vi "Motor_Temp_Monitor_V15.vi"() -> ()   [LabVIEW 2019]
uses:
  Instance           2 30Saved   Motor_Temp_Monitor_V11 .vi
  <vilib>/Utility/error.llb/DialogType.ctl
  Controls/Measurement Action.ctl
  <vilib>/ULx/Create Channel.llb/ULx Create Channel (DO-Digital Output).vi
  <vilib>/ULx/Write.llb/ULx Write (Digital Bool 1Line 1Point).vi
panel:
  out "Log Write":bool
  out "Cluster":T1 {"1" format="%.1f"; "11" format="%.1f"; "6" format="%.1f"; "9" format="%.1f"; "10" format="%.1f"; "15" format="%.1f"; "14" format="%.1f"; "13" format="%.1f"; "12" format="%.1f"; "5" format="%.1f"; "8" format="%.1f"; "2" format="%.1f"; "3" format="%.1f"; "4" format="%.1f"; "7" format="%.1f"}
  out "Stop Signal Status":bool
  in  "OK Button":bool
  out "Alarm":bool
  out "Alarm":bool
  in  "Motor Temp.\nLimit °C":sgl=60.0 min=0 max=200 step=1
  out "Time":string
  out "Date":string
  in  "Bearing Temp.\nLimit °C":sgl=40.0 min=0 max=200 step=1
  in  "stop":bool
  out "MOTOR TEMPERATURES\n[Deg C]":T2 caption="Motor Temperatures °C" {"6. Rear Motor: Armature Com End" format="%.1f"; "5. Rear Motor: Field Windings" format="%.1f"; "4. Rear Motor: Armature Ctr. Brg" format="%.1f"; "3. Front Motor: Armature Ctr. Brg" format="%.1f"; "1" format="%.1f"; "2\n2" format="%.1f"}
  in  "Tab Control":T3(tab)
  out "Motor Thermocouple Chart":waveform(dbl)[](graph)
  out "Motor Bearing Chart":waveform(dbl)[](graph)
  # "DOWTY PROPELLERS - WIND TUNNEL MOTOR TEMPERATURE MONITORING SYSTEM"
  # "V15.1 Ó2014 GE Aviation"
  # "M4"
  # "Motor Temperatures °C"
  # "M1"
  # "M2"
  # "M3"
  # "M4"
  # "M5"
  # "M6"
  # "2"
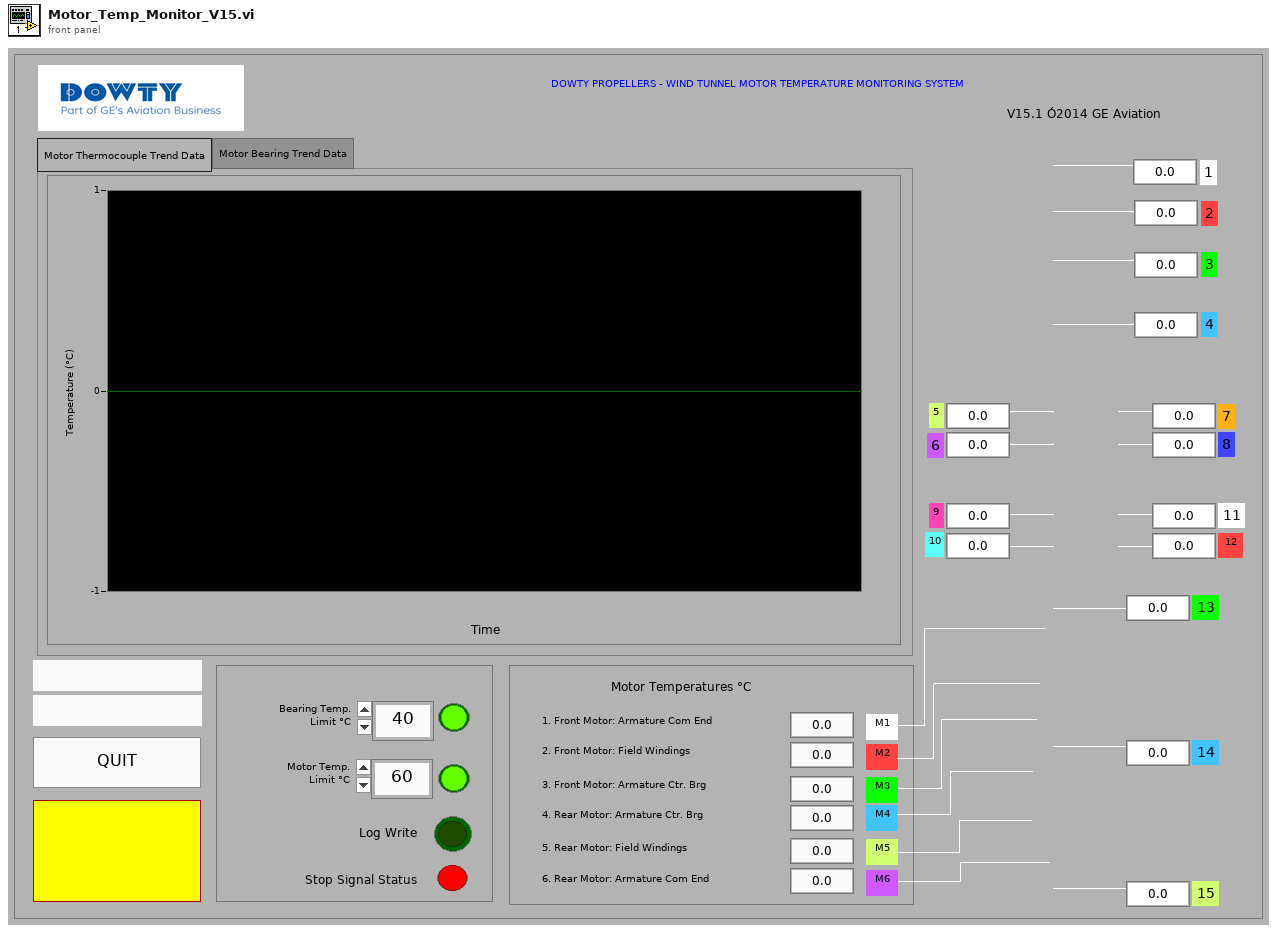
[diagram p1: front panel]
types:
  T1 = cluster{"1":sgl, "2":sgl, "3":sgl, "4":sgl, "5":sgl, "6":sgl, "7":sgl, "8":sgl, "9":sgl, "10":sgl, "11":sgl, "12":sgl, "13":sgl, "14":sgl, "15":sgl}
  T2 = cluster{"1":sgl, "2\n2":sgl, "3. Front Motor: Armature Ctr. Brg":sgl, "4. Rear Motor: Armature Ctr. Brg":sgl, "5. Rear Motor: Field Windings":sgl, "6. Rear Motor: Armature Com End":sgl}
  T3 = enum32{"Motor Thermocouple Trend Data", "Motor Bearing Trend Data"}
  T4 = typedef "Measurement Action.ctl" = enum16{"Open", "Read Bearing Temps", "Read Motor Temps", "Close"}
  T5 = enum16{"open", "replace", "create", "open or create", "replace or create", "replace or create with confirmation"}
  T6 = cluster{"second":i32, "minute":i32, "hour":i32, "day of month":i32, "month":i32, "year":i32, "day of week":i32, "day of year":i32, "is DST":i32}
  T7 = typedef "DialogType.ctl" = u16
  T8 = cluster{"Temps[0]":dbl, "Temps[1]":dbl, "Temps[2]":dbl, "Temps[3]":dbl, "Temps[4]":dbl, "Temps[5]":dbl}
  T9 = cluster{"Temps[0]":dbl, "Temps[1]":dbl, "Temps[2]":dbl, "Temps[3]":dbl, "Temps[4]":dbl, "Temps[5]":dbl, "Temps[6]":dbl, "Temps[7]":dbl, "Temps[8]":dbl, "Temps[9]":dbl, "Temps[10]":dbl, "Temps[11]":dbl, "Temps[12]":dbl, "Temps[13]":dbl, "Temps[14]":dbl}
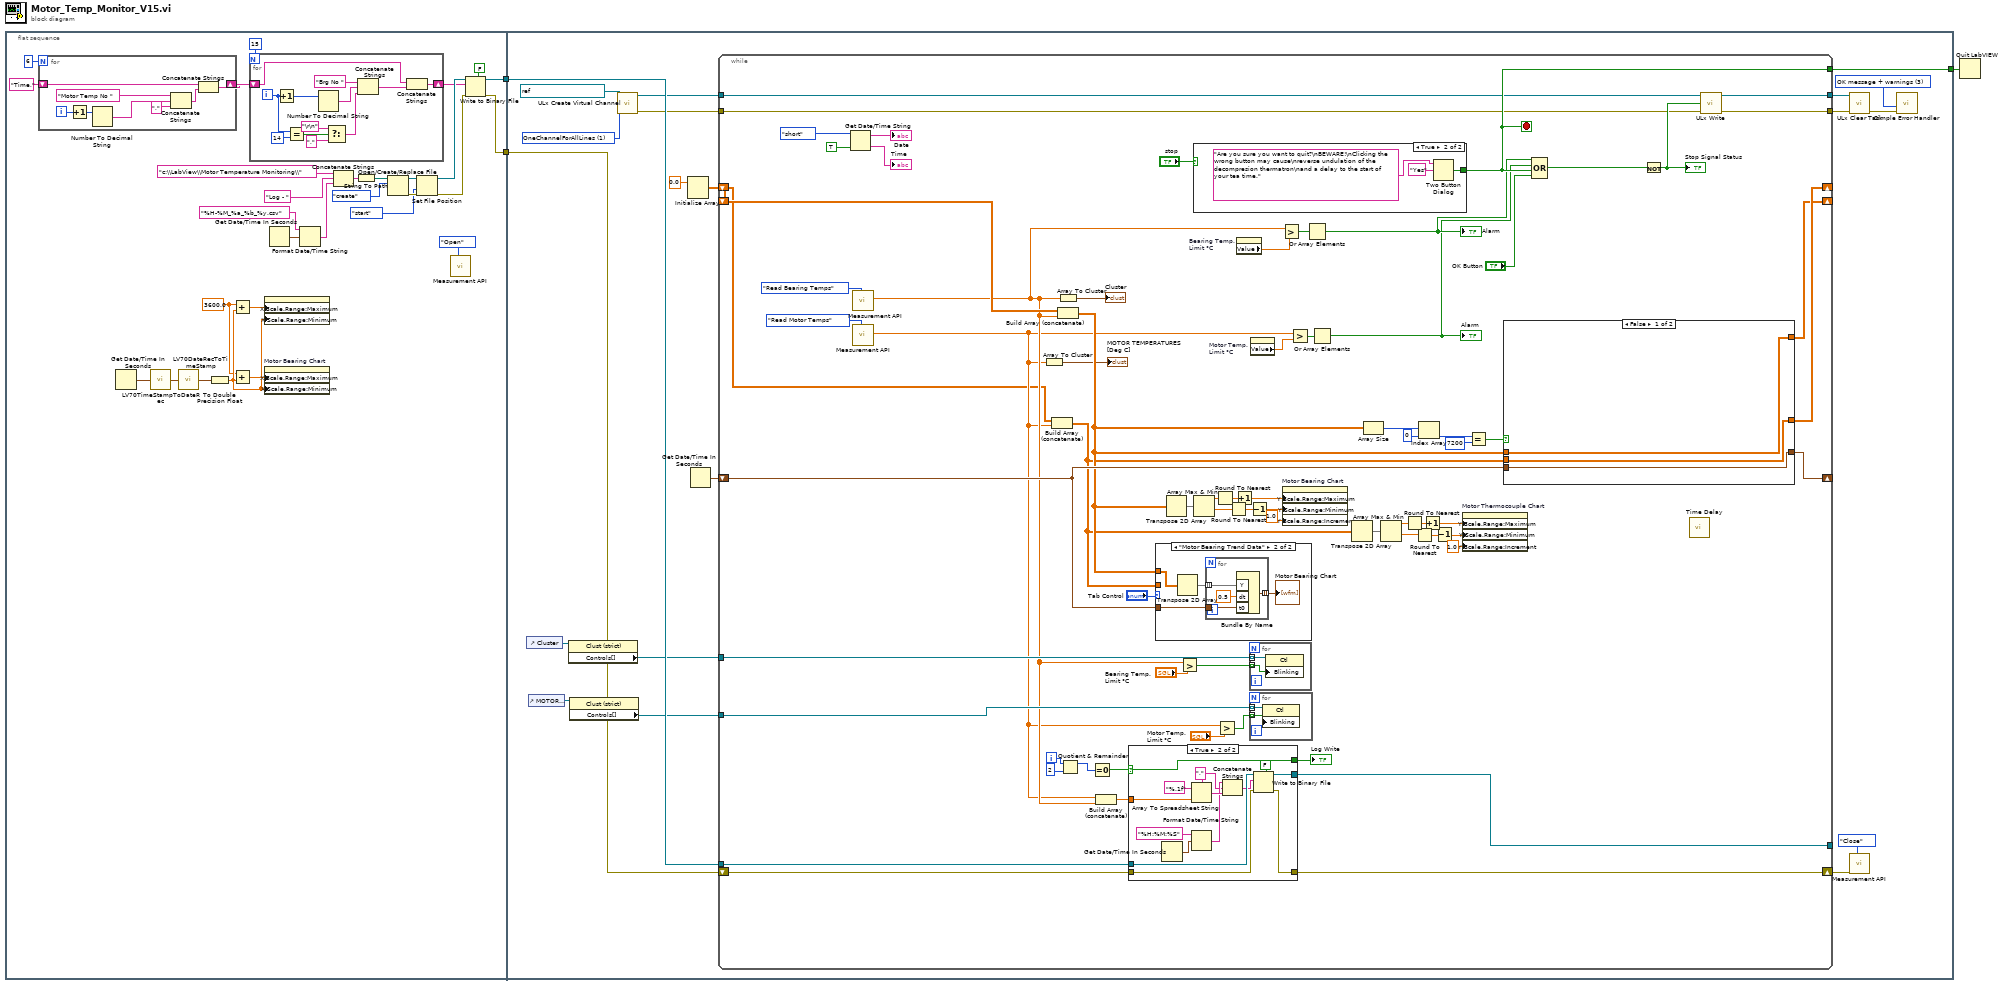
[diagram p0: block diagram]
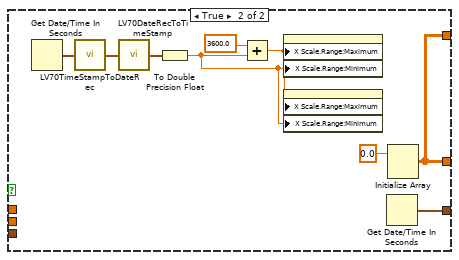
[diagram p4: hidden frame]
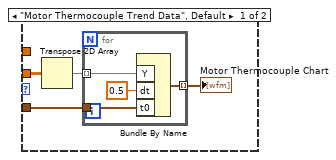
[diagram p5: hidden frame]
diagram:
  n1 = flat-sequence {
    tunnel: [w18] -> w2
    tunnel: [w16] -> w1
    tunnel: [w67] -> w3
    tunnel: w2 -> [w69]
    tunnel: w1 -> [w68]
    frame #0 {
      w27 = 3600.0
      n2 = for {
        N: 6 -> [_]
        shift-right: [w35] -> w5
        shift-left: "Time," -> [w37]
        i -> [w34]
        n3 = Increment(x=w34) -> (x+1=w40:i32)
        n4 = Number To Decimal String(number=w40) -> (decimal integer string=w38:string)  [unwired: 1 out]
        n5 = Concatenate Strings("Motor Temp No ", w38, ",") -> (w36:string)
        n6 = Concatenate Strings(w37, w36) -> (w35:string)
      }
      n7 = Get Date/Time In Seconds() -> (seconds since 1Jan1904=w8:timestamp)
      n8 = call <vilib>:"LV70TimeStampToDateRec.vi"("time stamp"=w8) -> ("date time rec"=w32:T6)
      n9 = call <vilib>:"LV70DateRecToTimeStamp.vi"("date time rec"=w32) -> ("Time Stamp"=w29:timestamp)
      n10 = To Double Precision Float(number=w29) -> (double precision float=w28:dbl)
      n11 = Add(x=w27, y=w28) -> (x+y=w30:dbl)
      n12 = Add(x=w27, y=w28) -> (x+y=w31:dbl)
      n13 = for {
        N: 15 -> [_]
        shift-right: [w47] -> w7
        shift-left: w5 -> [w49]
        i -> [w42]
        n14 = Increment(x=w42) -> (x+1=w52:i32)
        n15 = Equal?(x=w42, y=14) -> (x = y?=w44:bool)
        n16 = Number To Decimal String(number=w52) -> (decimal integer string=w50:string)  [unwired: 1 out]
        n17 = Select(t="\r\n", s=w44, f=",") -> (s? t:f=w41:string)
        n18 = Concatenate Strings("Brg No ", w50, w41) -> (w48:string)
        n19 = Concatenate Strings(w49, w48) -> (w47:string)
      }
      n20 = property on="Motor Thermocouple Chart" class="WFGraph (strict)"("X Scale.Range:Maximum"=w30, "X Scale.Range:Minimum"=w28) -> ()  [unwired: 2 in, 2 out]
      n21 = property on="Motor Bearing Chart" class="WFGraph (strict)"("X Scale.Range:Maximum"=w31, "X Scale.Range:Minimum"=w28) -> ()  [unwired: 2 in, 2 out]
      n22 = Get Date/Time In Seconds() -> (seconds since 1Jan1904=w21:timestamp)
      n23 = Format Date/Time String(time format string (%c)="%H-%M_%a_%b_%y.csv", seconds (now)=w21) -> (date/time string=w23:string)  [unwired: 1 out]
      n24 = Concatenate Strings("c:\\LabView\\Motor Temperature Monitoring\\", "Log - ", w23) -> (w26:string)
      n25 = String To Path(string=w26) -> (path=w20:path)
      n26 = Open/Create/Replace File(file path (use dialog)=w20, operation (0:open)=T5."create") -> (refnum out=w19:refnum<file>, error out=w17:errorcluster)  [unwired: 1 in, 4 out]
      n27 = Set File Position(refnum=w19, from (0:start)=enum16{"start", "end", "current"}."start" ("pos mode (0:2)"), error in=w17) -> (refnum out=w12:refnum<file>, error out=w11:errorcluster)  [unwired: 1 out]
      n28 = call "Measurement API.vi"("Action"=Measurement_Action."Open") -> ()  [unwired: 9 in, 2 out]
      n29 = Write to Binary File(file (use dialog)=w12, data=w7, error in=w11, 5:FALSE ("prepend array or string size? (T)")) -> (refnum out=w18:refnum<file>, error out=w16:errorcluster)  [unwired: 3 out]
    }
    frame #1 {
      w62 = 1 items=["OneChannelForEachLine", "OneChannelForAllLines"] ("line grouping")
      w59 = T7 3 items=["no dialog", "OK message", "continue or stop message", "OK message + warnings", "continue/stop + warnings"] ("type of dialog (OK msg:1)")
      n30 = control-ref of="Cluster"() -> (w58:refnum<vi>)
      n31 = control-ref of="MOTOR TEMPERATURES\n[Deg C]"() -> (w56:refnum<vi>)
      n32 = property class="Clust (strict)"(reference=w58) -> ("Controls[]"=w57:refnum<vi>[])  [unwired: 1 in, 2 out]
      n33 = property class="Clust (strict)"(reference=w56) -> ("Controls[]"=w55:refnum<vi>[])  [unwired: 1 in, 2 out]
      n34 = call-poly <vilib>:"ULx Create Virtual Channel.vi"("lines"=refnum<k21> "Dev0/AuxPort/Do0" ("Lines"), "line grouping"=w62) -> ("task out"=w61:refnum<k24>, "error out"=w60:errorcluster)  [unwired: 12 in]
      n35 = Initialize Array(0.0 ("element")) -> (w70:dbl[][])  [unwired: 2 out]
      n36 = Get Date/Time In Seconds() -> (seconds since 1Jan1904=w71:timestamp)
      n37 = while {
        shift-right: [w124] -> _
        shift-left: w70 -> [w74]
        shift-right: [w127] -> _
        shift-left: w71 -> [w126]
        shift-right: [w123] -> _
        shift-left: w70 -> [w128]
        tunnel: w69 -> [w105]
        shift-right: [w103] -> w54
        shift-left: w68 -> [w106]
        tunnel: [w104] -> _
        tunnel: [w94] -> w67
        tunnel: [w92] -> w65
        tunnel: [w91] -> w64
        tunnel: w61 -> [w90]
        tunnel: w60 -> [w89]
        tunnel: w57 -> [w79]
        tunnel: w55 -> [w80]
        i -> [w110]
        stop <- w94 stop-if-true
        n38 = Get Date/Time String(date format (0)=enum16{"short", "long", "abbreviated"}."short", want seconds? (F)=TRUE) -> (date string=→"Date":string, time string=→"Time":string)  [unwired: 1 out]
        n39 = call "Measurement API.vi"("Action"=Measurement_Action."Read Bearing Temps") -> ("Temps"=w77:dbl[])  [unwired: 9 in, 1 out]
        n40 = call "Measurement API.vi"("Action"=Measurement_Action."Read Motor Temps") -> ("Temps"=w75:dbl[])  [unwired: 9 in, 1 out]
        n41 = Array To Cluster(array=w75) -> (cluster=→"MOTOR TEMPERATURES\n[Deg C]":T8)
        n42 = Build Array (concatenate)(w74, w75) -> (w111:dbl[][])
        n43 = Array To Cluster(array=w77) -> (cluster=→"Cluster":T9)
        n44 = Build Array (concatenate)(w128, w77) -> (w116:dbl[][])
        n45 = Quotient & Remainder(x=w110, y=2) -> (x-y*floor(x/y)=w108:i32)  [unwired: 1 out]
        n46 = Equal To 0?(x=w108) -> (x = 0?=w107:bool)
        n47 = Build Array (concatenate)(w75, w77) -> (w81:dbl[])
        n48 = case shown="True" w107 {
          selector: w107 -> [_ w150]
          tunnel: w106 -> [w147 w160]
          tunnel: w105 -> [w148 w162]
          tunnel: [w148 w161] -> w104
          tunnel: [w147 w159] -> w103
          tunnel: w81 -> [_ w149]
          tunnel: [_ w150] -> w96
          frame False {
          }
          frame True {
            w152 = "," ("delimiter (Tab)")
            n49 = Get Date/Time In Seconds() -> (seconds since 1Jan1904=w157:timestamp)
            n50 = Array To Spreadsheet String(delimiter (Tab)=w152, array=w149, 3:"%.1f" ("format string")) -> (spreadsheet string=w155:string)
            n51 = Format Date/Time String(time format string (%c)="%H:%M:%S", seconds (now)=w157) -> (date/time string=w154:string)  [unwired: 1 out]
            n52 = Concatenate Strings(w154, w152, w155) -> (w153:string)
            n53 = Write to Binary File(file (use dialog)=w162, data=w153, error in=w160, 5:FALSE ("prepend array or string size? (T)")) -> (refnum out=w161:refnum<file>, error out=w159:errorcluster)  [unwired: 3 out]
          }
        }
        "Log Write" <- w96
        n54 = case shown="\"Motor Bearing Trend Data\"" "Tab Control" {
          tunnel: w126 -> [w178 w184]
          tunnel: w111 -> [w177 _]
          tunnel: w116 -> [_ w186]
          frame "Motor Thermocouple Trend Data", Default {
            n55 = Transpose 2D Array(2D array=w177) -> (transposed array=w176:dbl[][])
            n56 = for {
              tunnel: w176 -> [w179] mode=indexing
              tunnel: w178 -> [w181]
              tunnel: [w180] -> w175 mode=indexing
              n57 = Bundle By Name("Y"=w179, "dt"=0.5, "t0"=w181) -> (w180:waveform(dbl))  [unwired: 1 out]
            }
            "Motor Thermocouple Chart" <- w175
          }
          frame "Motor Bearing Trend Data" {
            n58 = Transpose 2D Array(2D array=w186) -> (transposed array=w185:dbl[][])
            n59 = for {
              tunnel: w185 -> [w187] mode=indexing
              tunnel: [w189] -> w183 mode=indexing
              tunnel: w184 -> [w188]
              n60 = Bundle By Name("Y"=w187, "dt"=0.5, "t0"=w188) -> (w189:waveform(dbl))  [unwired: 1 out]
            }
            "Motor Bearing Chart" <- w183
          }
        }
        n61 = Transpose 2D Array(2D array=w116) -> (transposed array=w115:dbl[][])
        n62 = Greater?(x=w77, y="Bearing Temp.\nLimit °C") -> (0:w139:bool[])
        n63 = case shown="True" "stop" {
          tunnel: [_ w146] -> w94
          frame False {
          }
          frame True {
            n64 = Two Button Dialog(message="Are you sure you want to quit?\nBEWARE!\nClicking the wrong button may cause\nreverse undulation of the decompresion thermatron\nand a delay to the start of your tea time.", 2:"Yes" ("T button name (\"OK\")")) -> (T button?=w146:bool)  [unwired: 1 out]
          }
        }
        n65 = Array Max & Min(array=w115) -> (max value=w114:dbl, min value=w113:dbl)  [unwired: 2 out]
        n66 = Round To Nearest(number=w114) -> (nearest integer value=w132:dbl)
        n67 = Greater?(x=w75, y="Motor Temp.\nLimit °C") -> (0:w102:bool[])
        n68 = Round To Nearest(number=w113) -> (nearest integer value=w133:dbl)
        n69 = Increment(x=w132) -> (x+1=w131:dbl)
        n70 = property on="Bearing Temp.\nLimit °C" class="DigNum (strict)"() -> ("Value"=w87:sgl)  [unwired: 2 in, 2 out]
        n71 = for {
          tunnel: w79 -> [w192] mode=indexing
          tunnel: w139 -> [w191] mode=indexing
          n72 = property class="Ctl"(reference=w192, "Blinking"=w191) -> ()  [unwired: 1 in, 2 out]
        }
        n73 = for {
          tunnel: w80 -> [w194] mode=indexing
          tunnel: w102 -> [w193] mode=indexing
          n74 = property class="Ctl"(reference=w194, "Blinking"=w193) -> ()  [unwired: 1 in, 2 out]
        }
        n75 = Decrement(x=w133) -> (x-1=w130:dbl)
        n76 = property on="Motor Temp.\nLimit °C" class="DigNum (strict)"() -> ("Value"=w73:sgl)  [unwired: 2 in, 2 out]
        n77 = Greater?(x=w77, y=w87) -> (0:w88:bool[])
        n78 = property on="Motor Bearing Chart" class="WFGraph (strict)"("Y Scale.Range:Maximum"=w131, "Y Scale.Range:Minimum"=w130, "Y Scale.Range:Increment"=1.0) -> ()  [unwired: 2 in, 2 out]
        n79 = Greater?(x=w75, y=w73) -> (0:w85:bool[])
        n80 = Or Array Elements(Boolean array=w88) -> (logical OR=w86:bool)
        "Alarm" <- w86
        n81 = Or Array Elements(Boolean array=w85) -> (logical OR=w84:bool)
        "Alarm" <- w84
        n82 = Transpose 2D Array(2D array=w111) -> (transposed array=w112:dbl[][])
        n83 = Array Size(array=w116) -> (size(s)=w121:i32[])
        n84 = Array Max & Min(array=w112) -> (max value=w118:dbl, min value=w117:dbl)  [unwired: 2 out]
        n85 = Round To Nearest(number=w118) -> (nearest integer value=w138:dbl)
        n86 = Round To Nearest(number=w117) -> (nearest integer value=w136:dbl)
        n87 = Index Array(array=w121, index=0) -> (element=w120:i32)
        n88 = Increment(x=w138) -> (x+1=w137:dbl)
        n89 = Decrement(x=w136) -> (x-1=w135:dbl)
        n90 = property on="Motor Thermocouple Chart" class="WFGraph (strict)"("Y Scale.Range:Maximum"=w137, "Y Scale.Range:Minimum"=w135, "Y Scale.Range:Increment"=1.0) -> ()  [unwired: 2 in, 2 out]
        n91 = Equal?(x=w120, y=7200) -> (x = y?=w125:bool)
        n92 = case shown="False" w125 {
          tunnel: [w164 w170] -> w124
          tunnel: [w165 w173] -> w127
          tunnel: w126 -> [w165 _]
          tunnel: w111 -> [w164 _]
          tunnel: w116 -> [w163 _]
          tunnel: [w163 w170] -> w123
          frame False {
          }
          frame True {
            n93 = Get Date/Time In Seconds() -> (seconds since 1Jan1904=w166:timestamp)
            n94 = call <vilib>:"LV70TimeStampToDateRec.vi"("time stamp"=w166) -> ("date time rec"=w172:T6)
            n95 = call <vilib>:"LV70DateRecToTimeStamp.vi"("date time rec"=w172) -> ("Time Stamp"=w171:timestamp)
            n96 = To Double Precision Float(number=w171) -> (double precision float=w168:dbl)
            n97 = Add(x=3600.0, y=w168) -> (x+y=w169:dbl)
            n98 = property on="Motor Bearing Chart" class="WFGraph (strict)"("X Scale.Range:Maximum"=w169, "X Scale.Range:Minimum"=w168) -> ()  [unwired: 2 in, 2 out]
            n99 = property on="Motor Thermocouple Chart" class="WFGraph (strict)"("X Scale.Range:Maximum"=w169, "X Scale.Range:Minimum"=w168) -> ()  [unwired: 2 in, 2 out]
            n100 = Get Date/Time In Seconds() -> (seconds since 1Jan1904=w173:timestamp)
            n101 = Initialize Array(0.0 ("element")) -> (w170:dbl[][])  [unwired: 2 out]
          }
        }
        n102 = Compound Arithmetic op=OR(w86, w84, w94, "OK Button") -> (w98:bool)
        n103 = Not(x=w98) -> (.not. x?=w93:bool)
        "Stop Signal Status" <- w93
        n104 = call "Time Delay"() -> ()  [unwired: 2 in, 10 out]
        n105 = call-poly <vilib>:"ULx Write.vi"("task in"=w90, "data"=w93, "error in"=w89) -> ("task out"=w92:refnum<k24>, "error out"=w91:errorcluster)  [unwired: 10 in, 1 out]
      }
      n106 = call <vilib>:"ULx Clear Task.vi"("task in"=w65, "error in"=w64) -> ("error out"=w66:errorcluster)  [unwired: 13 in]
      n107 = call "Measurement API.vi"("Action"=Measurement_Action."Close", "error IO"=w54) -> ()  [unwired: 8 in, 2 out]
      n108 = call <vilib>:"Simple Error Handler.vi"("type of dialog (OK msg:1)"=w59, "error in (no error)"=w66) -> ()  [unwired: 3 in, 5 out]
    }
  }
  n109 = Quit LabVIEW(quit? (T)=w3) -> ()
